vi "SSL Detection Frame.vi"(4 "ignora esquerda?":bool, 6 "ignora direita?":bool, 8 "error in":errorcluster, 9 "Array":u8[](array[numeric]) format="%02x") -> (0 "error out":errorcluster, 3 "Detection Frame":T1 {"robots_blue"."height" format="%+4.3f"; "robots_blue"."pixel_y" format="%+4.3f"; "robots_blue"."pixel_x" format="%+4.3f"; "robots_blue"."orientation" format="%+4.3f"; "robots_blue"."y" format="%+4.3f"; "robots_blue"."confidence" format="%4.3f"; "robots_blue"."x" format="%+4.3f"; "robots_yellow"."height" format="%+4.3f"; "robots_yellow"."pixel_y" format="%+4.3f"; "robots_yellow"."pixel_x" format="%+4.3f"; "robots_yellow"."orientation" format="%+4.3f"; "robots_yellow"."y" format="%+4.3f"; "robots_yellow"."confidence" format="%4.3f"; "robots_yellow"."x" format="%+4.3f"})   [LabVIEW 2023]
uses:
  Controls/SSL Detection Frame.ctl
  Controls/SSL Detection Robot.ctl
  <vilib>/Analysis/Matrix/Datatypes/RealMatrix.ctl
  Controls/SSL Detection Ball.ctl
  Varint Decoder uint32.vi
  <vilib>/Analysis/Matrix/NI_Matrix.lvlib
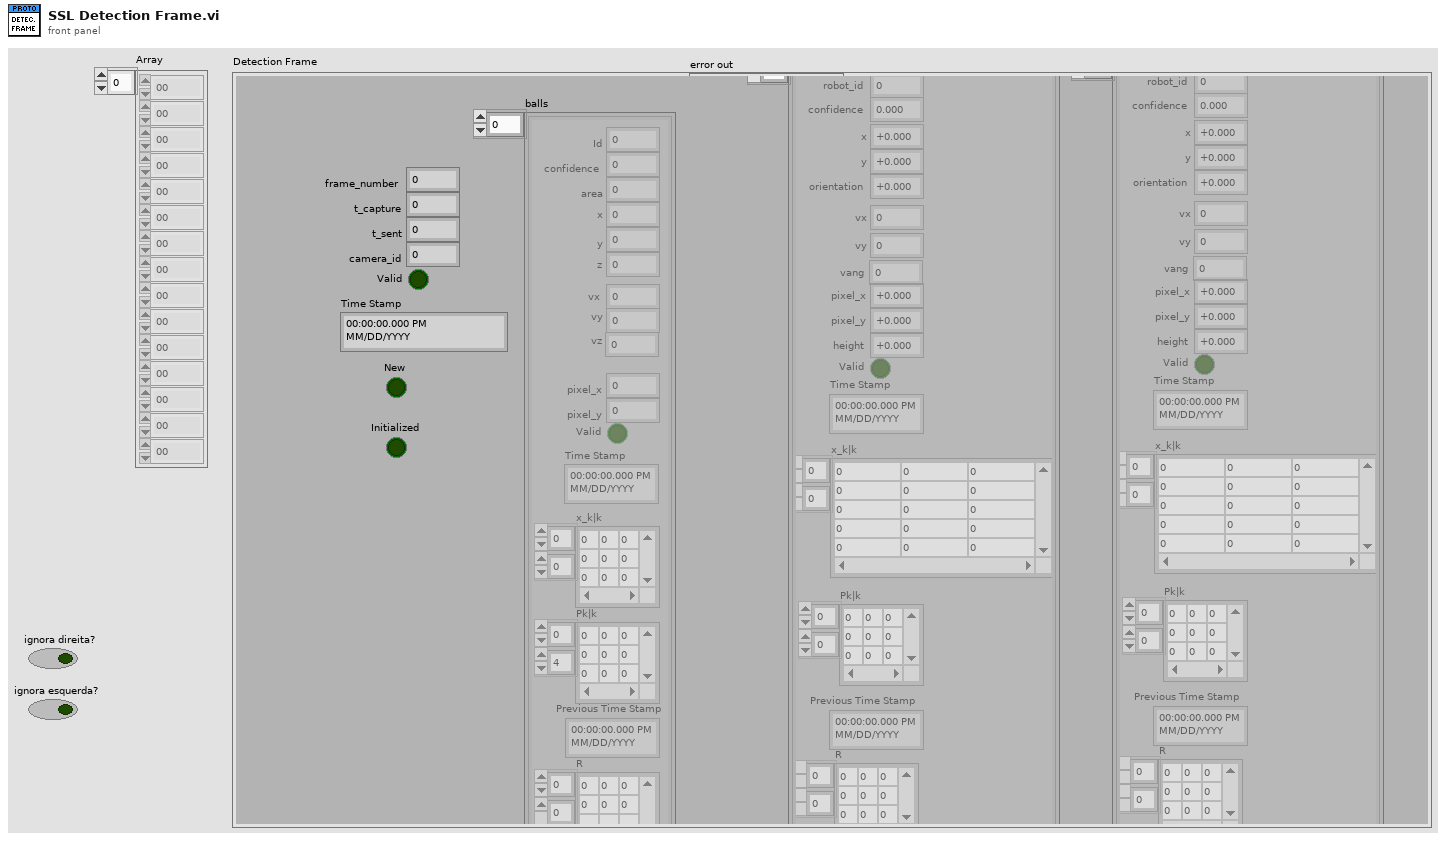
[diagram p1: front panel]
types:
  T1 = typedef "SSL Detection Frame.ctl" = cluster{"frame_number":u32, "t_capture":dbl, "t_sent":dbl, "camera_id":u32, "robots_yellow":T2[], "robots_blue":T2[], "balls":T4[], "Valid":bool, "Time Stamp":timestamp, "New":bool, "Initialized":bool}
  T2 = typedef "SSL Detection Robot.ctl" = cluster{"x":sgl, "robot_id":u32, "confidence":sgl, "y":sgl, "orientation":sgl, "pixel_x":sgl, "pixel_y":sgl, "height":sgl, "Valid":bool, "Time Stamp":timestamp, "x_k|k":T3, "Pk|k":T3, "Previous Time Stamp":timestamp, "R":T3, "vx":dbl, "vy":dbl, "vang":dbl}
  T3 = typedef "NI_Matrix.lvlib/RealMatrix.ctl" = dbl[][]
  T4 = typedef "SSL Detection Ball.ctl" = cluster{"x":sgl, "area":u32, "confidence":sgl, "y":sgl, "z":sgl, "pixel_x":sgl, "pixel_y":sgl, "Valid":bool, "Time Stamp":timestamp, "x_k|k":T3, "Pk|k":T3, "Id":u32, "Previous Time Stamp":timestamp, "R":T3, " vx":sgl, "vy":dbl, "vz":dbl}
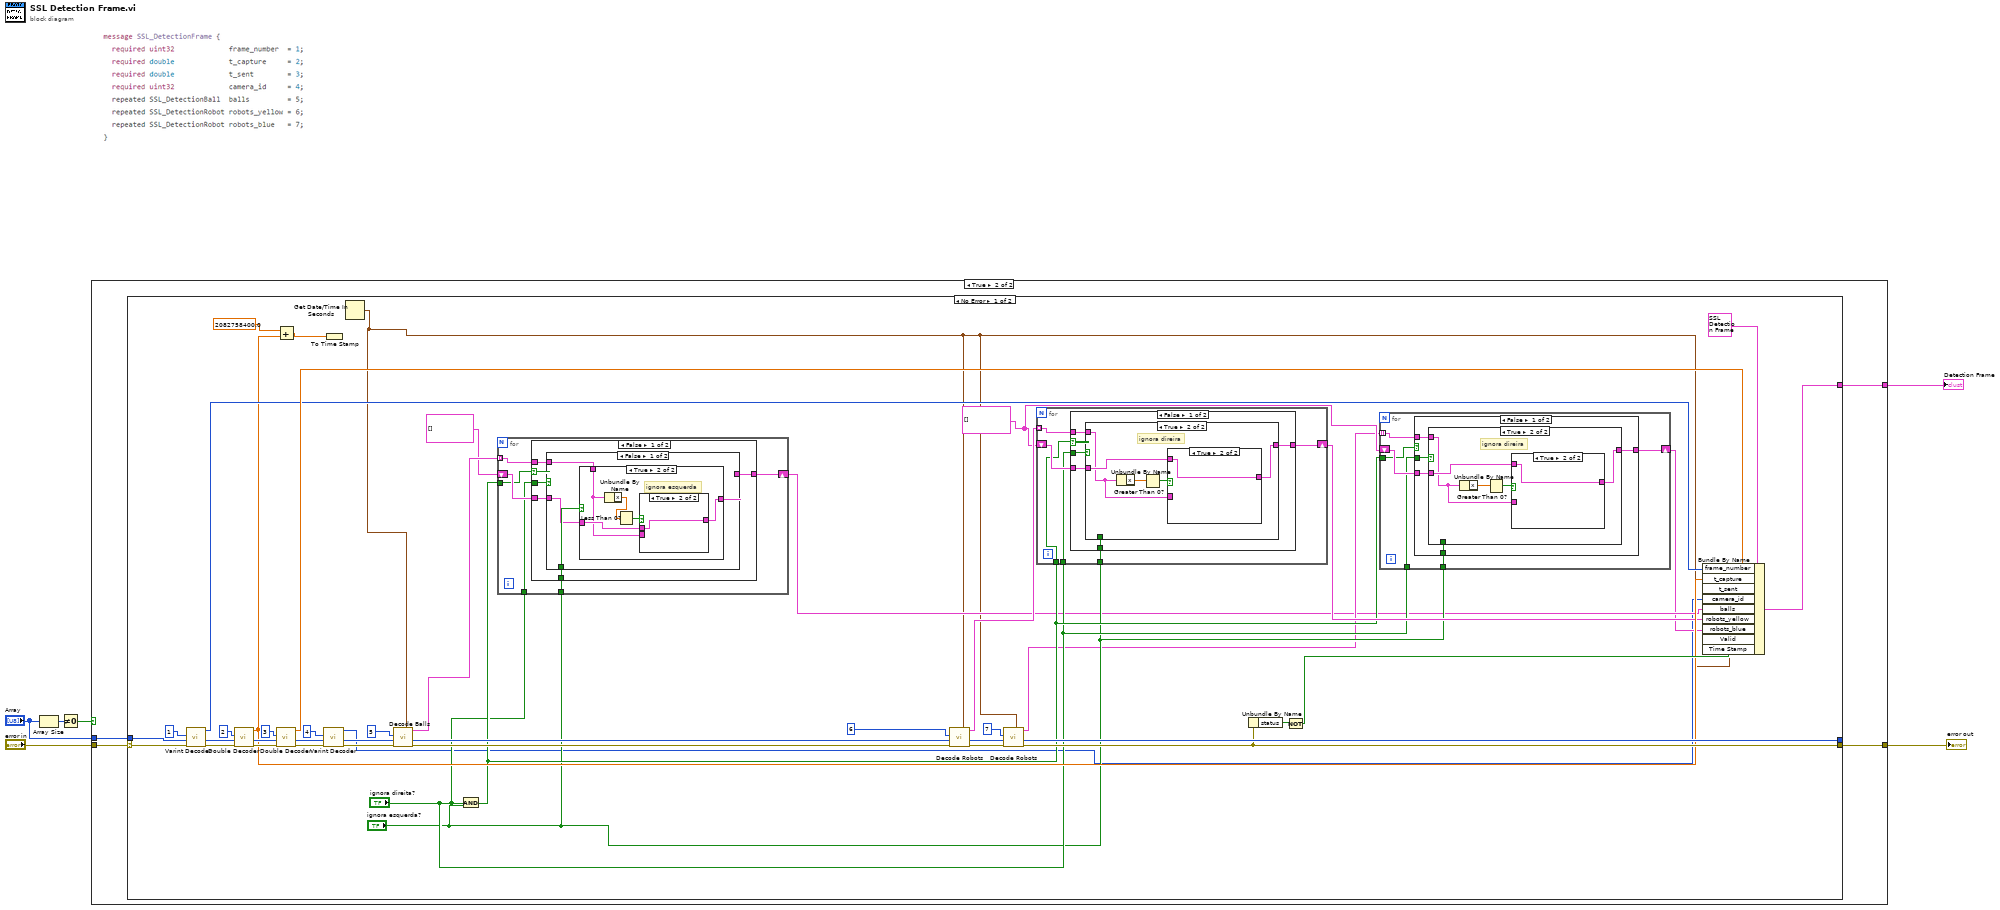
[diagram p0: block diagram]
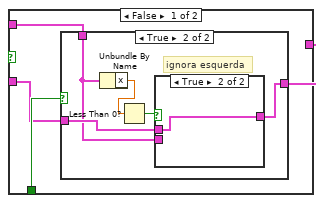
[diagram p3: hidden frame]
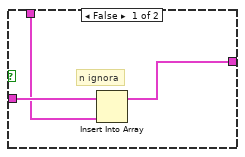
[diagram p4: hidden frame]
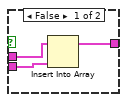
[diagram p5: hidden frame]
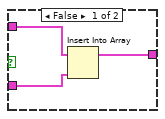
[diagram p6: hidden frame]
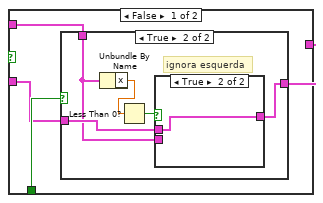
[diagram p8: hidden frame]
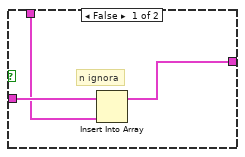
[diagram p9: hidden frame]
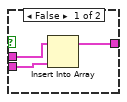
[diagram p10: hidden frame]
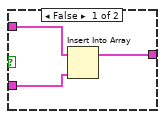
[diagram p11: hidden frame]
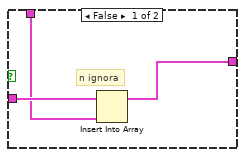
[diagram p13: hidden frame]
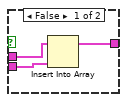
[diagram p14: hidden frame]
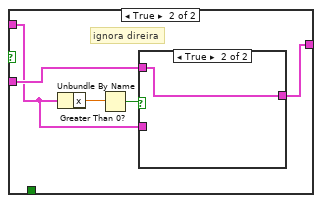
[diagram p15: hidden frame]
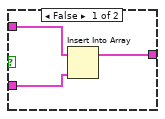
[diagram p16: hidden frame]
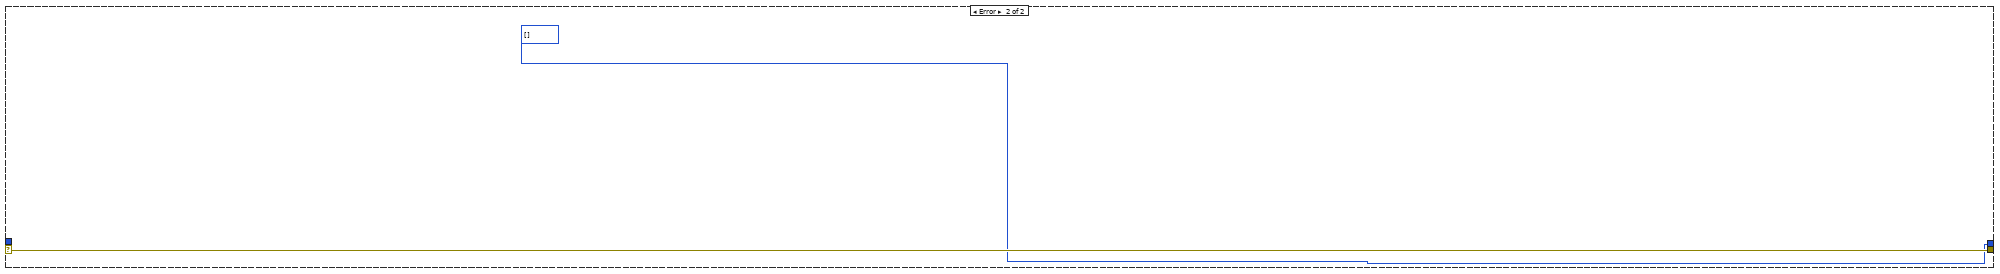
[diagram p18: hidden frame]
diagram:
  n1 = Array Size(array="Array") -> (size(s)=w4:i32)
  n2 = Not Equal To 0?(x=w4) -> (x != 0?=w2:bool)
  n3 = case shown="True" w2 {
    tunnel: "error in" -> [_ w10]
    tunnel: "Array" -> [_ w9]
    tunnel: [_ w8] -> w3
    tunnel: [_ w7] -> w1
    frame False {
    }
    frame True {
      n4 = case shown="No Error" w10 {
        selector: w10 -> [w54 w168]
        tunnel: [w30 w168] -> w8
        tunnel: [w32 u8[] [] ("array w/ subset deleted")] -> _
        tunnel: w9 -> [w31 _]
        tunnel: [w27 _] -> w7
        frame No Error {
          w16 = T2[] [] ("Robots")
          n5 = call-poly "Varint Decoder.vi"("error in (no error)"=w54, "Array"=w31, "Key"=1) -> ("error out"=w53:errorcluster, "array w/ subset deleted"=w40:u8[], "Varint"=w44:u32)  [unwired: 5 in, 1 out]
          n6 = call "Double Decoder.vi"("error in (no error)"=w53, "Array"=w40, "Key"=2) -> ("error out"=w52:errorcluster, "array w/ subset deleted"=w41:u8[], "Double"=w26:dbl)  [unwired: 5 in, 1 out]
          n7 = call "Double Decoder.vi"("error in (no error)"=w52, "Array"=w41, "Key"=3) -> ("error out"=w51:errorcluster, "array w/ subset deleted"=w42:u8[], "Double"=w45:dbl)  [unwired: 5 in, 1 out]
          n8 = Add(x=2082758400.0, y=w26) -> (x+y=w24:dbl)
          n9 = call-poly "Varint Decoder.vi"("error in (no error)"=w51, "Array"=w42, "Key"=4) -> ("error out"=w47:errorcluster, "array w/ subset deleted"=w43:u8[], "Varint"=w11:u32)  [unwired: 5 in, 1 out]
          n10 = To Time Stamp(1:w24) -> ()  [unwired: 1 out]
          n11 = Get Date/Time In Seconds() -> (seconds since 1Jan1904=w13:timestamp)
          n12 = call "Decode Balls.vi"("Time Stamp"=w13, "error in"=w47, "array"=w43, "Key"=5) -> ("error out"=w38:errorcluster, "array w/ subset deleted out"=w37:u8[], "Array"=w23:T4[])  [unwired: 5 in]
          n13 = And(x="ignora direita?", y="ignora esquerda?") -> (x .and. y?=w20:bool)
          n14 = for {
            tunnel: w23 -> [w133] mode=indexing
            tunnel: "ignora direita?" -> [w131]
            shift-right: [w135] -> w14
            shift-left: T4[] [] ("Array") -> [w132]
            tunnel: w20 -> [w130]
            tunnel: "ignora esquerda?" -> [w134]
            n15 = case shown="False" w130 {
              tunnel: [w138 w166] -> w135
              tunnel: w131 -> [w140 _]
              tunnel: w134 -> [w139 _]
              tunnel: w133 -> [w137 _]
              tunnel: w132 -> [w136 w166]
              frame False {
                n16 = case shown="False" w140 {
                  tunnel: w139 -> [w144 _]
                  tunnel: [w143 w157] -> w138
                  tunnel: w137 -> [w142 w158]
                  tunnel: w136 -> [w141 w159]
                  frame False {
                    n17 = case shown="True" w144 {
                      tunnel: [w147 w148] -> w143
                      tunnel: w142 -> [w145 w149]
                      tunnel: w141 -> [w146 w150]
                      frame False {
                        # "n ignora"
                        n18 = Insert Into Array(array=w146, new element=w145) -> (w147:T4[])  [unwired: 1 in]
                      }
                      frame True {
                        # "ignora esquerda"
                        n19 = Unbundle By Name(w149) -> ("x"=w151:sgl)
                        n20 = Less Than 0?(x=w151) -> (x < 0?=w152:bool)
                        n21 = case shown="True" w152 {
                          tunnel: w150 -> [w155 w156]
                          tunnel: w149 -> [w154 _]
                          tunnel: [w153 w156] -> w148
                          frame False {
                            n22 = Insert Into Array(array=w155, new element=w154) -> (w153:T4[])  [unwired: 1 in]
                          }
                          frame True {
                          }
                        }
                      }
                    }
                  }
                  frame True {
                    # "ignora direira"
                    n23 = Unbundle By Name(w158) -> ("x"=w160:sgl)
                    n24 = Greater Than 0?(x=w160) -> (x > 0?=w161:bool)
                    n25 = case shown="True" w161 {
                      tunnel: w159 -> [w164 w165]
                      tunnel: w158 -> [w163 _]
                      tunnel: [w162 w165] -> w157
                      frame False {
                        n26 = Insert Into Array(array=w164, new element=w163) -> (w162:T4[])  [unwired: 1 in]
                      }
                      frame True {
                      }
                    }
                  }
                }
              }
              frame True {
              }
            }
          }
          n27 = call "Decode Robots.vi"("Time Stamp"=w13, "error in"=w38, "array"=w37, "Key"=6) -> ("error out"=w35:errorcluster, "array w/ subset deleted out"=w34:u8[], "Robots"=w17:T2[])  [unwired: 5 in]
          n28 = call "Decode Robots.vi"("Time Stamp"=w13, "error in"=w35, "array"=w34, "Key"=7) -> ("error out"=w30:errorcluster, "array w/ subset deleted out"=w32:u8[], "Robots"=w15:T2[])  [unwired: 5 in]
          n29 = for {
            tunnel: w17 -> [w96] mode=indexing
            tunnel: "ignora direita?" -> [w93]
            shift-right: [w98] -> w21
            shift-left: w16 -> [w95]
            tunnel: "ignora esquerda?" -> [w97]
            tunnel: w20 -> [w94]
            n30 = case shown="False" w94 {
              tunnel: [w101 w129] -> w98
              tunnel: w93 -> [w103 _]
              tunnel: w97 -> [w102 _]
              tunnel: w96 -> [w100 _]
              tunnel: w95 -> [w99 w129]
              frame False {
                n31 = case shown="True" w103 {
                  tunnel: w102 -> [w107 _]
                  tunnel: [w106 w120] -> w101
                  tunnel: w100 -> [w105 w121]
                  tunnel: w99 -> [w104 w122]
                  frame False {
                    n32 = case shown="True" w107 {
                      tunnel: [w110 w111] -> w106
                      tunnel: w105 -> [w108 w112]
                      tunnel: w104 -> [w109 w113]
                      frame False {
                        # "n ignora"
                        n33 = Insert Into Array(array=w109, new element=w108) -> (w110:T2[])  [unwired: 1 in]
                      }
                      frame True {
                        # "ignora esquerda"
                        n34 = Unbundle By Name(w112) -> ("x"=w114:sgl)
                        n35 = Less Than 0?(x=w114) -> (x < 0?=w115:bool)
                        n36 = case shown="True" w115 {
                          tunnel: w113 -> [w118 w119]
                          tunnel: w112 -> [w117 _]
                          tunnel: [w116 w119] -> w111
                          frame False {
                            n37 = Insert Into Array(array=w118, new element=w117) -> (w116:T2[])  [unwired: 1 in]
                          }
                          frame True {
                          }
                        }
                      }
                    }
                  }
                  frame True {
                    # "ignora direira"
                    n38 = Unbundle By Name(w121) -> ("x"=w123:sgl)
                    n39 = Greater Than 0?(x=w123) -> (x > 0?=w124:bool)
                    n40 = case shown="True" w124 {
                      tunnel: w122 -> [w127 w128]
                      tunnel: w121 -> [w126 _]
                      tunnel: [w125 w128] -> w120
                      frame False {
                        n41 = Insert Into Array(array=w127, new element=w126) -> (w125:T2[])  [unwired: 1 in]
                      }
                      frame True {
                      }
                    }
                  }
                }
              }
              frame True {
              }
            }
          }
          n42 = Unbundle By Name(w30) -> ("status"=w29:bool)
          n43 = Not(x=w29) -> (.not. x?=w28:bool)
          n44 = for {
            tunnel: w15 -> [w59] mode=indexing
            tunnel: "ignora direita?" -> [w57]
            shift-right: [w61] -> w12
            shift-left: w16 -> [w58]
            tunnel: w20 -> [w56]
            tunnel: "ignora esquerda?" -> [w60]
            n45 = case shown="False" w56 {
              tunnel: [w64 w92] -> w61
              tunnel: w57 -> [w66 _]
              tunnel: w60 -> [w65 _]
              tunnel: w59 -> [w63 _]
              tunnel: w58 -> [w62 w92]
              frame False {
                n46 = case shown="True" w66 {
                  tunnel: w65 -> [w70 _]
                  tunnel: [w69 w83] -> w64
                  tunnel: w63 -> [w68 w84]
                  tunnel: w62 -> [w67 w85]
                  frame False {
                    n47 = case shown="True" w70 {
                      tunnel: [w73 w74] -> w69
                      tunnel: w68 -> [w71 w75]
                      tunnel: w67 -> [w72 w76]
                      frame False {
                        # "n ignora"
                        n48 = Insert Into Array(array=w72, new element=w71) -> (w73:T2[])  [unwired: 1 in]
                      }
                      frame True {
                        # "ignora esquerda"
                        n49 = Unbundle By Name(w75) -> ("x"=w77:sgl)
                        n50 = Less Than 0?(x=w77) -> (x < 0?=w78:bool)
                        n51 = case shown="True" w78 {
                          tunnel: w76 -> [w81 w82]
                          tunnel: w75 -> [w80 _]
                          tunnel: [w79 w82] -> w74
                          frame False {
                            n52 = Insert Into Array(array=w81, new element=w80) -> (w79:T2[])  [unwired: 1 in]
                          }
                          frame True {
                          }
                        }
                      }
                    }
                  }
                  frame True {
                    # "ignora direira"
                    n53 = Unbundle By Name(w84) -> ("x"=w86:sgl)
                    n54 = Greater Than 0?(x=w86) -> (x > 0?=w87:bool)
                    n55 = case shown="True" w87 {
                      tunnel: w85 -> [w90 w91]
                      tunnel: w84 -> [w89 _]
                      tunnel: [w88 w91] -> w83
                      frame False {
                        n56 = Insert Into Array(array=w90, new element=w89) -> (w88:T2[])  [unwired: 1 in]
                      }
                      frame True {
                      }
                    }
                  }
                }
              }
              frame True {
              }
            }
          }
          n57 = Bundle By Name(cluster=T1 {"frame_number"=0, "t_capture"=0.0, "t_sent"=0.0, "camera_id"=0, "robots_yellow"=[], "robots_blue"=[], "balls"=[], "Valid"=FALSE, "Time Stamp"=timestamp(0 s since 1904-01-01), "New"=FALSE, "Initialized"=FALSE} ("Detection Frame 2"), "frame_number"=w44, "t_capture"=w26, "t_sent"=w45, "camera_id"=w11, "balls"=w14, "robots_yellow"=w21, "robots_blue"=w12, "Valid"=w28, "Time Stamp"=w13) -> (w27:T1)
        }
        frame Error {
        }
      }
    }
  }
  "error out" <- w3
  "Detection Frame" <- w1
